vi "initialise_image_aquisition.vi"(7 "Imaging Variables In":T1={"Region of interest"=[], "Number of buffers"=0, "Frame timeout (ms)"=1000}) -> (2 "New Image Array":T2[](array[typedef]), 4 "IMAQ Session Out":refnum<k11>, 8 "Imaging Variables Out":T1={"Region of interest"=[], "Number of buffers"=0, "Frame timeout (ms)"=1000}, 15 "error out":errorcluster)   [LabVIEW 2023]
uses:
  <vilib>/vision/Image Controls.llb/IMAQ Image.ctl
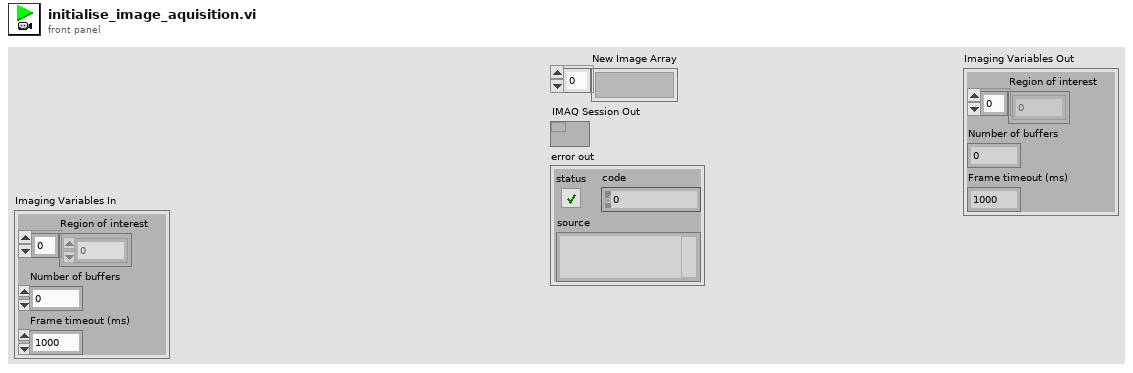
[diagram p1: front panel]
types:
  T1 = cluster{"Region of interest":i32[], "Number of buffers":u32, "Frame timeout (ms)":u32}
  T2 = typedef "IMAQ Image.ctl" = refnum<image>
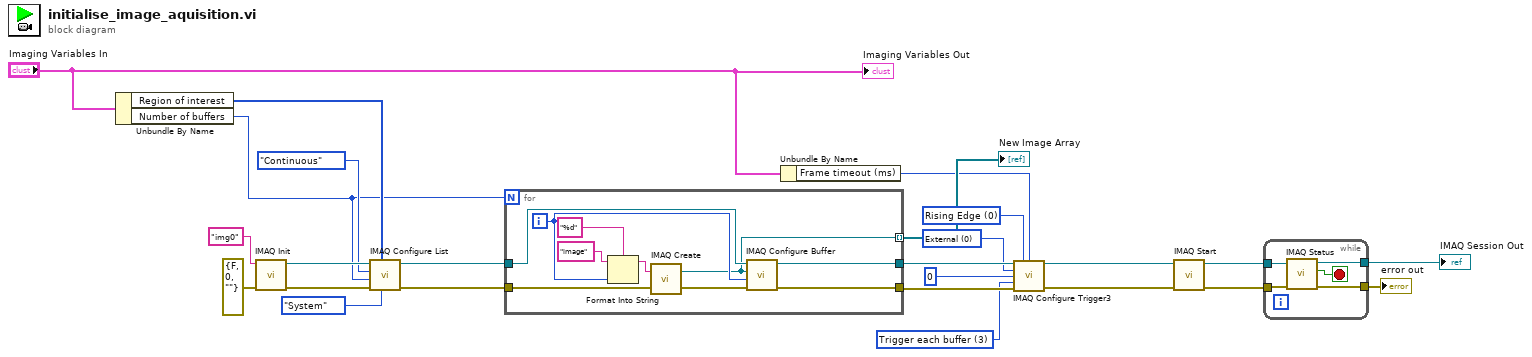
[diagram p0: block diagram]
diagram:
  w13 = u32 3 items=["Disabled", "Trigger start of acquisition", "Trigger start of each buffer list", "Trigger each buffer", "Trigger each line (linescan)", "Trigger end of acquisition"] ("Action")
  w14 = u32 0 items=["Rising Edge", "Falling Edge"] ("Polarity")
  w15 = u32 0 items=["External"=0, "RTSI"=1, "ISO In"=2, "Scaled Encoder"=5, "Software Trigger"=6] ("Type")
  n1 = Unbundle By Name("Imaging Variables In") -> ("Region of interest"=w4:i32[], "Number of buffers"=w3:u32)
  n2 = call <vilib>:"IMAQ Init.vi"("error in (no error)"=errorcluster {"status"=FALSE, "code"=0, "source"=""}, "Interface Name"="img0") -> ("error out"=w23:errorcluster, "IMAQ Session Out"=w24:refnum<k11>)  [unwired: 8 in]
  n3 = call <vilib>:"IMAQ Configure List.vi"("Memory Location"=enum16{"System", "Onboard"}."System", "Region of interest"=w4, "error in (no error)"=w23, "Number of buffers"=w3, "Continuous?"=enum16{"One-Shot", "Continuous"}."Continuous", "IMAQ Session In"=w24) -> ("error out"=w18:errorcluster, "IMAQ Session Out"=w19:refnum<k11>)  [unwired: 4 in]
  n4 = for {
    N: w3 -> [_]
    tunnel: [w35] -> w17
    tunnel: [w34] -> w16
    tunnel: w19 -> [w33]
    tunnel: w18 -> [w29]
    tunnel: [w26] -> w7 mode=indexing
    i -> [w27]
    n5 = Format Into String(format string="%d", initial string="image", w27) -> (resulting string=w30:string)  [unwired: 1 in, 1 out]
    n6 = call "IMAQ Create"("Image Name"=w30, "error in (no error)"=w29) -> ("New Image"=w26:T2, "error out"=w28:errorcluster)  [unwired: 3 in]
    n7 = call <vilib>:"IMAQ Configure Buffer.vi"("error in (no error)"=w28, "Buffer Number"=w27, "Image In"=w26, "IMAQ Session In"=w33) -> ("error out"=w34:errorcluster, "IMAQ Session Out"=w35:refnum<k11>)  [unwired: 6 in]
  }
  "New Image Array" <- w7
  n8 = Unbundle By Name("Imaging Variables In") -> ("Frame timeout (ms)"=w2:u32)
  n9 = call <vilib>:"IMAQ Configure Trigger3.vi"("IMAQ Session In"=w17, "Polarity"=w14, "Frame timeout (ms)"=w2, "Type"=w15, "Line Number"=u32 0, "Action"=w13, "error in (no error)"=w16) -> ("IMAQ Session Out"=w11:refnum<k11>, "error out"=w10:errorcluster)  [unwired: 7 in]
  n10 = call <vilib>:"IMAQ Start.vi"("error in (no error)"=w10, "IMAQ Session In"=w11) -> ("error out"=w8:errorcluster, "IMAQ Session Out"=w9:refnum<k11>)  [unwired: 8 in]
  n11 = while {
    tunnel: w9 -> [w40]
    tunnel: w8 -> [w39]
    tunnel: [w37] -> w6
    tunnel: [w36] -> w5
    stop <- w38 stop-if-true
    n12 = call <vilib>:"IMAQ Status.vi"("error in (no error)"=w39, "IMAQ Session In"=w40) -> ("error out"=w36:errorcluster, "Acquiring?"=w38:bool, "IMAQ Session Out"=w37:refnum<k11>)  [unwired: 5 in, 2 out]
  }
  "IMAQ Session Out" <- w6
  "error out" <- w5
  "Imaging Variables Out" <- "Imaging Variables In"
